vi "Console.vi"() -> ()   [LabVIEW 2017]
uses:
  Print Options.ctl
panel:
  out "Console Out":string
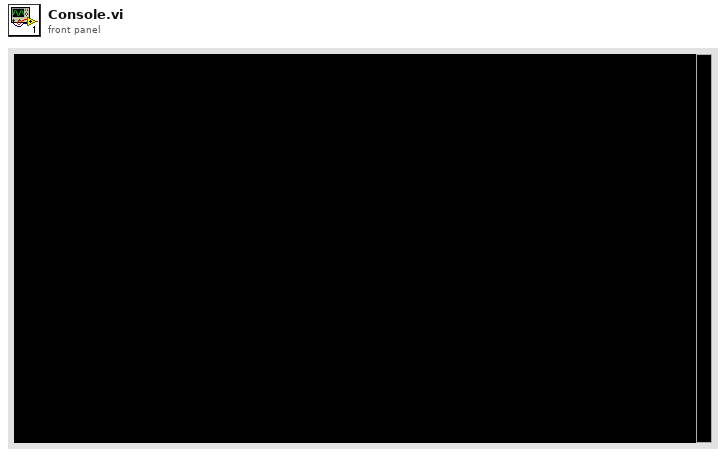
[diagram p1: front panel]
types:
  T1 = typedef "Print Options.ctl" = enum16{"Create", "Get Reference", "Print", "Print Header", "Close"}
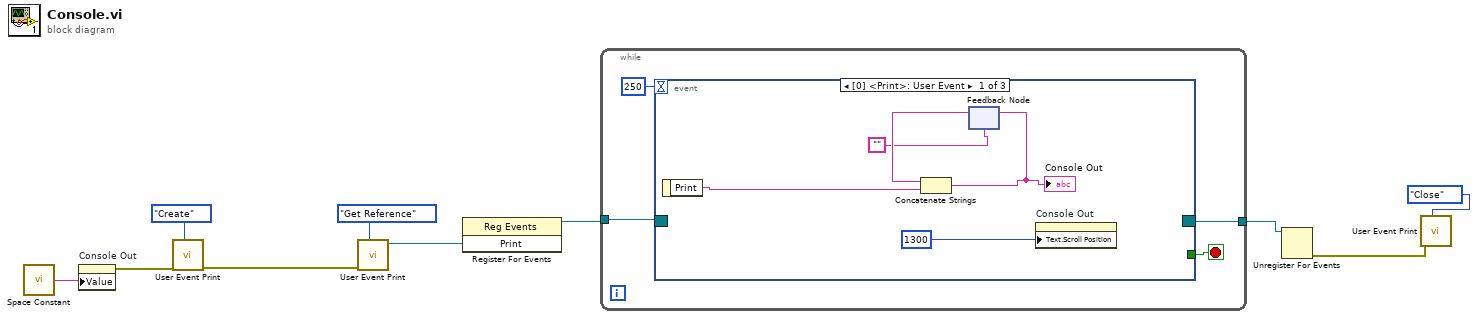
[diagram p0: block diagram]
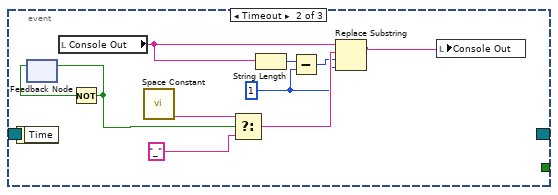
[diagram p2: hidden frame]
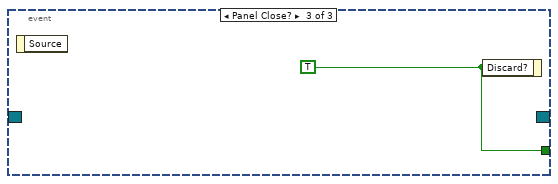
[diagram p3: hidden frame]
diagram:
  n1 = call <vilib>:"Space Constant.vi"() -> ("String"=w1:string)
  n2 = property on="Console Out" class="Str"("Value"=w1) -> (error out=w2:errorcluster)  [unwired: 2 in, 1 out]
  n3 = call "User Event Print.vi"("Options"=Print_Options."Create", "error in (no error)"=w2) -> ("error out"=w4:errorcluster)  [unwired: 8 in, 1 out]
  n4 = call "User Event Print.vi"("Options"=Print_Options."Get Reference", "error in (no error)"=w4) -> ("Print"=w3:refnum<user-event>)  [unwired: 8 in, 1 out]
  n5 = register-events(w3) -> (reference out=w9:refnum<event-registration>)  [unwired: 2 in, 1 out]
  n6 = while {
    tunnel: w9 -> [w13]
    tunnel: [w12] -> w10
    stop <- w14 stop-if-true
    n7 = event shown="[0] <Print>: User Event" {
      selector: w13 -> [_ _ _]
      dyn-events: [_ _ _] -> w12
      timeout: 250 -> [_ _ _]
      tunnel: [_ _ w30] -> w14
      event User Event {
        n8 = event-data() -> ("Print"=w19:string)  [unwired: 1 in]
        n9 = feedback #1("") -> (w18:string)
        n10 = Concatenate Strings(w18, w19) -> (w16:string)
        "Console Out" <- w16
        n11 = feedback-in #1(w16) -> ()
        n12 = property on="Console Out" class="Str"("Text.Scroll Position"=u32 1300) -> ()  [unwired: 2 in, 2 out]
      }
      event Timeout {
        w22 = 1 ("length (len. of substring)")
        n13 = event-data() -> ()  [unwired: 1 in, 1 out]
        n14 = feedback #2() -> (w29:bool)  [unwired: 1 in]
        n15 = local read "Console Out"() -> (w27:string)
        n16 = Not(x=w29) -> (.not. x?=w26:bool)
        n17 = feedback-in #2(w26) -> ()
        n18 = call <vilib>:"Space Constant.vi"() -> ("String"=w21:string)
        n19 = Select(t=w21, s=w26, f="_") -> (s? t:f=w25:string)
        n20 = String Length(string=w27) -> (length=w24:i32)
        n21 = Subtract(x=w24, y=w22) -> (x-y=w23:i32)
        n22 = Replace Substring(2:w22, 3:w23, 4:w25, 5:w27) -> (1:w28:string)  [unwired: 1 out]
        n23 = local write "Console Out"(w28) -> ()
      }
      event Panel Close? {
        w30 = TRUE ("Discard?")
        n24 = event-data() -> ()  [unwired: 1 in, 1 out]
        n25 = event-data("Discard?"=w30) -> ()  [unwired: 1 in, 1 out]
      }
    }
  }
  n26 = Unregister For Events(event registration refnum=w10) -> (error out=w8:errorcluster)  [unwired: 1 in]
  n27 = call "User Event Print.vi"("Options"=Print_Options."Close", "error in (no error)"=w8) -> ()  [unwired: 8 in, 2 out]
